vi "Close.vi"(8 "error in (no error)":errorcluster, 11 "RP Communicator in":refnum<class "RP Communicator.lvclass">) -> (0 "error out":errorcluster, 3 "RP Communicator out":refnum<class "RP Communicator.lvclass">)   [LabVIEW 2015, in "RP Communicator.lvclass"]
uses:
  RP Communicator.lvclass
  RP Command.ctl
  RP Communicator.lvclass/RP Communicator.ctl
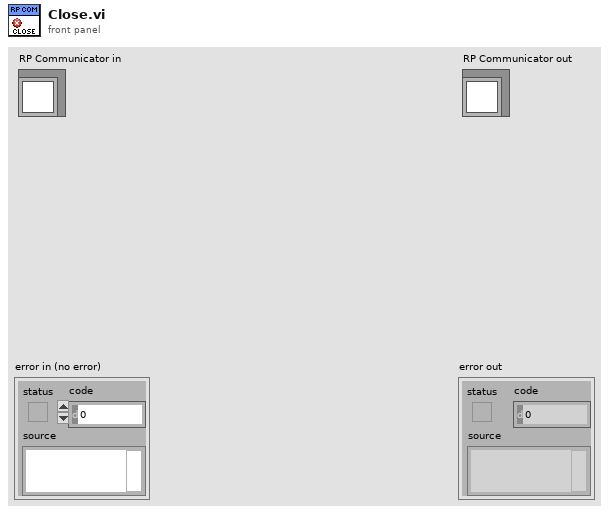
[diagram p1: front panel]
types:
  T1 = typedef "RP Command.ctl" = enum16{"Reset", "Read IDN", "Stop server", "Get status", "Get temperature", "Connect client", "Arm", "Software trigger", "Get whole buffer", "Get chunk", "System call", "Get config", "Set config", "Recieve data", "Play pattern", "Transmit data"}
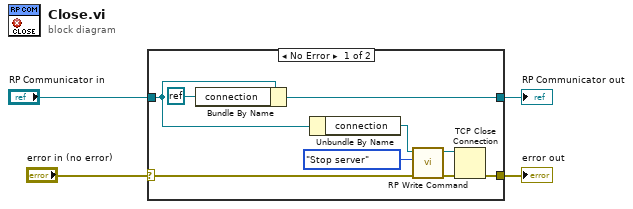
[diagram p0: block diagram]
diagram:
  n1 = case shown="No Error" "error in (no error)" {
    selector: "error in (no error)" -> [w10 w15]
    tunnel: [w5 w15] -> w3
    tunnel: [w7 w14] -> w1
    tunnel: "RP Communicator in" -> [w13 w14]
    frame No Error {
      n2 = Bundle By Name(cluster=w13, "connection"=refnum<k0> refnum) -> (w7:refnum<class "RP Communicator.lvclass">)
      n3 = Unbundle By Name(w13) -> ("connection"=w12:refnum<k5>)
      n4 = call "RP Write Command.vi"("Error In"=w10, "Command number"=RP_Command."Stop server", "connection ID"=w12) -> ("Error Out"=w9:errorcluster, "connection ID out"=w8:refnum<k5>)  [unwired: 6 in, 1 out]
      n5 = TCP Close Connection(connection ID=w8, error in (no error)=w9) -> (error out=w5:errorcluster)  [unwired: 1 in, 1 out]
    }
    frame Error {
    }
  }
  "error out" <- w3
  "RP Communicator out" <- w1
